vi "Find Theta.vi"(10 "X":dbl, 11 "Y":dbl) -> (3 "Theta":dbl)   [LabVIEW 2014]
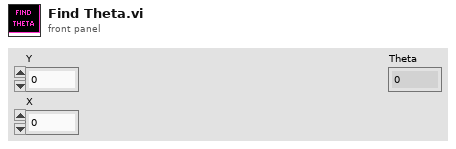
[diagram p1: front panel]
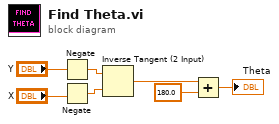
[diagram p0: block diagram]
diagram:
  n1 = Negate(x="Y") -> (-x=w4:dbl)
  n2 = Negate(x="X") -> (-x=w5:dbl)
  n3 = Inverse Tangent (2 Input)(1:w5, 2:w4) -> (0:w6:dbl)
  n4 = Add(x=w6, y=180.0) -> (x+y=→"Theta":dbl)
